vi "Write Skills.vi"(8 "error in (no error)":errorcluster, 10 "Skills":T1, 11 "KickTactic in":refnum<class "KickTactic.lvclass">) -> (0 "error out":errorcluster, 3 "KickTactic out":refnum<class "KickTactic.lvclass">)   [LabVIEW 2023, in "KickTactic.lvclass"]
uses:
  KickTactic.lvclass
  KickToSkill_v2_class/KickToSkill_v2.lvclass
  Circulate_class/CirculateSkill.lvclass
  AlignSkill/AlignSkill.lvclass
  KickTactic.lvclass/KickTactic.ctl
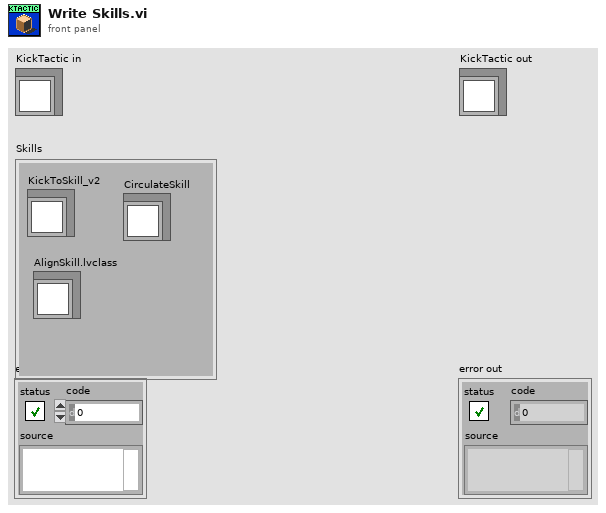
[diagram p1: front panel]
types:
  T1 = cluster{"KickToSkill_v2":refnum<class "KickToSkill_v2.lvclass">, "CirculateSkill":refnum<class "CirculateSkill.lvclass">, "AlignSkill.lvclass":refnum<class "AlignSkill.lvclass">}
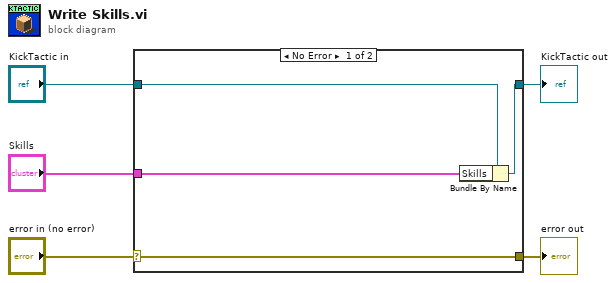
[diagram p0: block diagram]
diagram:
  n1 = case shown="No Error" "error in (no error)" {
    selector: "error in (no error)" -> [w9 w10]
    tunnel: [w9 w10] -> w4
    tunnel: [w7 w11] -> w2
    tunnel: "KickTactic in" -> [w8 w11]
    tunnel: "Skills" -> [w6 _]
    frame No Error {
      n2 = Bundle By Name(cluster=w8, "Skills"=w6) -> (w7:refnum<class "KickTactic.lvclass">)
    }
    frame Error {
    }
  }
  "error out" <- w4
  "KickTactic out" <- w2
